vi "Scripting_Example.vi"   [LabVIEW 2017, in "labview-standard-library.lvlib" / "automode-scripting.lvlib"]
uses:
  automode-scripting.lvlib
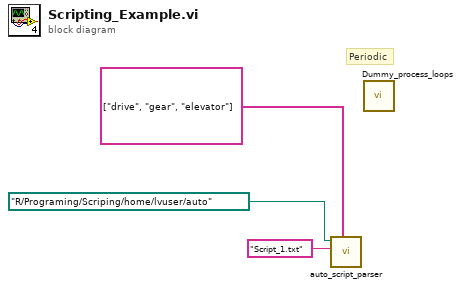
[diagram p0: block diagram]
diagram:
  # "Periodic"
  n1 = call "auto_script_parser.vi"("Process notifier names"=string[] ["drive", "gear", "elevator"], "Script name in"="Script_1.txt", "Script folder path"=path "R:/Programing/Scriping/home/lvuser/auto" ("Path")) -> ()  [unwired: 9 in]
  n2 = call "Dummy_process_loops.vi"() -> ()  [unwired: 12 in]
